vi "Launch Nested.vi"(8 "error in (no error)":errorcluster, 9 "Config Element":refnum<class "VolatusConfigElement.lvclass">, 10 "Nested Module":refnum<class "Module.lvclass">, 11 "Parent in":refnum<class "Module.lvclass">) -> (0 "error out":errorcluster, 2 "MessageQ":refnum<class "MessageQ.lvclass">, 3 "Parent out":refnum<class "Module.lvclass">)   [LabVIEW 2020, in "Volatus.lvlib" / "Module.lvclass"]
uses:
  Module.lvclass
  MessageQ/MessageQ.lvclass
  Module.lvclass/Module.ctl
  VolatusConfig/VolatusConfigElement/VolatusConfigElement.lvclass
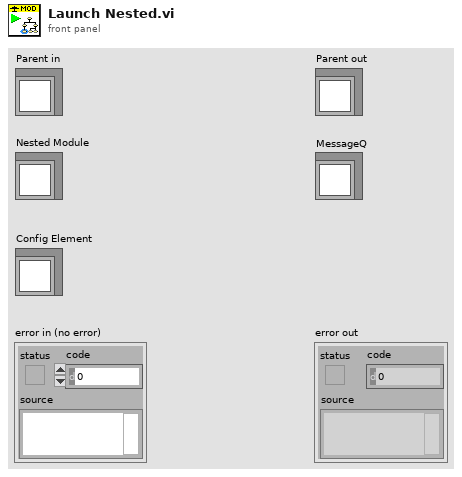
[diagram p1: front panel]
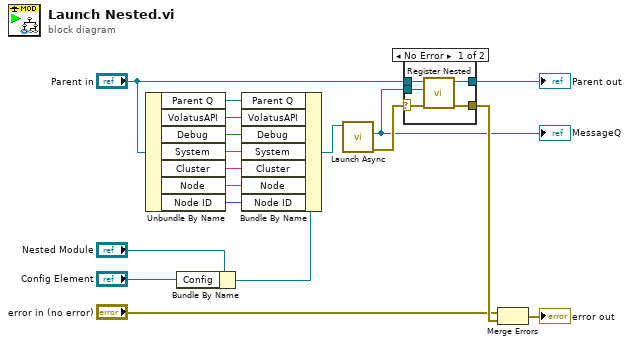
[diagram p0: block diagram]
diagram:
  n1 = Unbundle By Name("Parent in") -> ("Parent Q"=w10:refnum<class "MessageQ.lvclass">, "VolatusAPI"=w9:refnum<class "VolatusAPI.lvclass">, "Debug"=w5:bool, "System"=w4:string, "Cluster"=w3:string, "Node"=w2:string, "Node ID"=w1:u32)
  n2 = Bundle By Name(cluster="Nested Module", "Config"="Config Element") -> (w7:refnum<class "Module.lvclass">)
  n3 = Bundle By Name(cluster=w7, "Parent Q"=w10, "VolatusAPI"=w9, "Debug"=w5, "System"=w4, "Cluster"=w3, "Node"=w2, "Node ID"=w1) -> (w14:refnum<class "Module.lvclass">)
  n4 = call "Launch Async.vi"("Module in"=w14) -> ("error out"=w17:errorcluster, "MessageQ"=w8:refnum<class "MessageQ.lvclass">)  [unwired: 9 in]
  "MessageQ" <- w8
  n5 = case shown="No Error" w17 {
    selector: w17 -> [w21 w24]
    tunnel: w8 -> [w22 _]
    tunnel: "Parent in" -> [w23 w25]
    tunnel: [w19 w25] -> w12
    tunnel: [w20 w24] -> w18
    frame No Error {
      n6 = call "Register Nested.vi"("error in (no error)"=w21, "MessageQ"=w22, "Module in"=w23) -> ("error out"=w20:errorcluster, "Module out"=w19:refnum<class "Module.lvclass">)  [unwired: 7 in]
    }
    frame Error {
    }
  }
  "Parent out" <- w12
  n7 = Merge Errors("error in (no error)", w18) -> (→"error out":errorcluster)
